vi "Send Command.vi"(8 "error in":errorcluster, 9 "Value":variant, 10 "Command":string, 11 "Electronic Load in":refnum<class "Electronic Load.lvclass">) -> (0 "error out":errorcluster, 3 "Electronic Load out":refnum<class "Electronic Load.lvclass">)   [LabVIEW 2019, in "Electronic Load.lvlib" / "Electronic Load.lvclass"]
uses:
  Library/Electronic Load.lvclass
  C:/Users/Public/Documents/Development/builds/Engine/Engine.lvlibp/Project/Engine.lvclass
  Electronic Load Messages/Write OCP Delay Msg/Write OCP Delay Msg.lvclass/Write OCP Delay Msg.ctl
  Electronic Load Messages/Write OCP Enable Msg/Write OCP Enable Msg.lvclass/Write OCP Enable Msg.ctl
  Electronic Load Messages/Write OCP Level Msg/Write OCP Level Msg.lvclass/Write OCP Level Msg.ctl
  Electronic Load Messages/Write Active Channel Msg/Write Active Channel Msg.lvclass/Write Active Channel Msg.ctl
  Electronic Load Messages/Write Input Level Msg/Write Input Level Msg.lvclass/Write Input Level Msg.ctl
  Electronic Load Messages/Write Mode Msg/Write Mode Msg.lvclass/Write Mode Msg.ctl
  Electronic Load Messages/Write Output Enable Msg/Write Output Enable Msg.lvclass/Write Output Enable Msg.ctl
  Electronic Load Messages/Write Slew Rate Msg/Write Slew Rate Msg.lvclass/Write Slew Rate Msg.ctl
  Electronic Load Messages/Write All Pulse Msg/Write All Pulse Msg.lvclass/Write All Pulse Msg.ctl
  Electronic Load Messages/Write Pulse Data Points Msg/Write Pulse Data Points Msg.lvclass/Write Pulse Data Points Msg.ctl
  Electronic Load Messages/Write Pulse Delay Msg/Write Pulse Delay Msg.lvclass/Write Pulse Delay Msg.ctl
  Electronic Load Messages/Write Pulse Enable Msg/Write Pulse Enable Msg.lvclass/Write Pulse Enable Msg.ctl
  Electronic Load Messages/Write Pulse Initial Msg/Write Pulse Initial Msg.lvclass/Write Pulse Initial Msg.ctl
  Electronic Load Messages/Write Pulse Mode Msg/Write Pulse Mode Msg.lvclass/Write Pulse Mode Msg.ctl
  Electronic Load Messages/Write Pulse Sample Interval Msg/Write Pulse Sample Interval Msg.lvclass/Write Pulse Sample Interval Msg.ctl
  Electronic Load Messages/Write Pulse Slew Msg/Write Pulse Slew Msg.lvclass/Write Pulse Slew Msg.ctl
  Electronic Load Messages/Write Pulse Width Msg/Write Pulse Width Msg.lvclass/Write Pulse Width Msg.ctl
  Electronic Load Messages/Write Transient Msg/Write Transient Msg.lvclass/Write Transient Msg.ctl
  builds/Engine/Engine.lvlibp/Accessors/Read Self Q.vi
  builds/Engine/Actor Framework.lvlibp/1abvi3w/vi.lib/ActorFramework/Message Enqueuer/Enqueue.vi
  builds/Engine/Actor Framework.lvlibp/1abvi3w/vi.lib/ActorFramework/Message Enqueuer/Message Enqueuer.lvclass
  Electronic Load Messages/Write OCP Delay Msg/Write OCP Delay Msg.lvclass
  Electronic Load Messages/Write OCP Enable Msg/Write OCP Enable Msg.lvclass
  Electronic Load Messages/Write OCP Level Msg/Write OCP Level Msg.lvclass
  Electronic Load Messages/Write Active Channel Msg/Write Active Channel Msg.lvclass
  Electronic Load Messages/Write Input Level Msg/Write Input Level Msg.lvclass
  Electronic Load Messages/Write Mode Msg/Write Mode Msg.lvclass
  Electronic Load Messages/Write Output Enable Msg/Write Output Enable Msg.lvclass
  Electronic Load Messages/Write Slew Rate Msg/Write Slew Rate Msg.lvclass
  Electronic Load Messages/Write All Pulse Msg/Write All Pulse Msg.lvclass
  Electronic Load Messages/Write Pulse Data Points Msg/Write Pulse Data Points Msg.lvclass
  Electronic Load Messages/Write Pulse Delay Msg/Write Pulse Delay Msg.lvclass
  Electronic Load Messages/Write Pulse Enable Msg/Write Pulse Enable Msg.lvclass
  Electronic Load Messages/Write Pulse Initial Msg/Write Pulse Initial Msg.lvclass
  Electronic Load Messages/Write Pulse Mode Msg/Write Pulse Mode Msg.lvclass
  Electronic Load Messages/Write Pulse Sample Interval Msg/Write Pulse Sample Interval Msg.lvclass
  Electronic Load Messages/Write Pulse Slew Msg/Write Pulse Slew Msg.lvclass
  Electronic Load Messages/Write Pulse Width Msg/Write Pulse Width Msg.lvclass
  Electronic Load Messages/Write Transient Msg/Write Transient Msg.lvclass
  Electronic Load Messages/Reset Eload Msg/Reset Eload Msg.lvclass
  builds/Instruments/Instruments.lvlibp/Instruments Messages/Take Snapshot Msg/Take Snapshot Msg.lvclass
  builds/Instruments/Instruments.lvlibp/Instruments Messages/Power Off Msg/Power Off Msg.lvclass
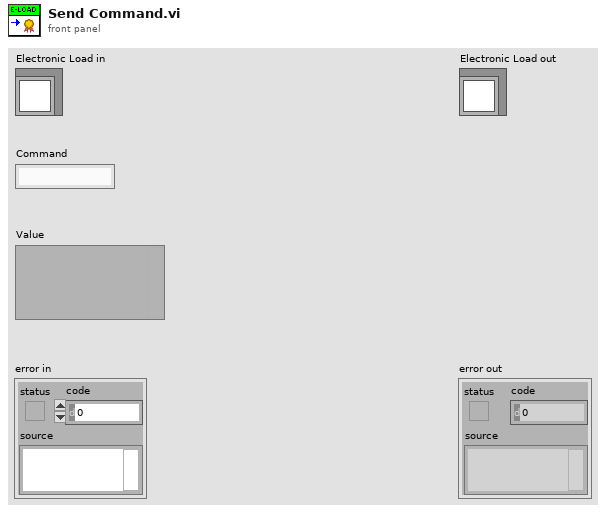
[diagram p1: front panel]
types:
  T1 = typedef "Electronic Load.lvlib/Electronic Load.lvclass/E-Load Mode.ctl" = enum16{"Current", "Resistance", "Voltage"}
  T2 = typedef "Electronic Load.lvlib/Electronic Load.lvclass/Trigger Settings.ctl" = cluster{"Mode":T1, "Initial":dbl, "Transient":dbl, "Interval":dbl, "Width":dbl, "Delay":dbl, "Data Pts":i32, "Slew Rate":dbl}
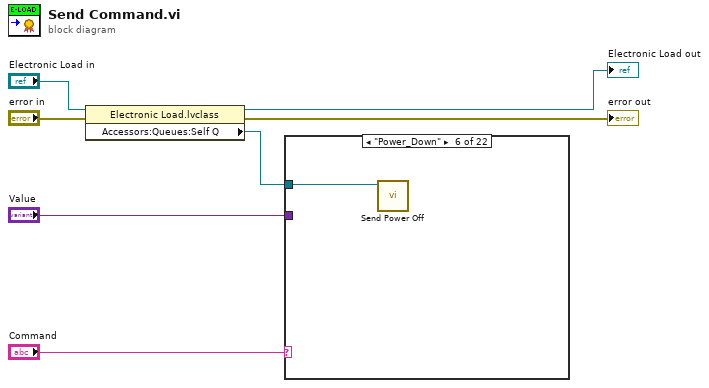
[diagram p0: block diagram]
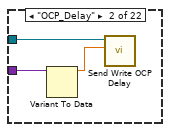
[diagram p3: hidden frame]
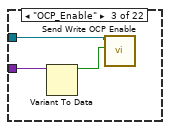
[diagram p4: hidden frame]
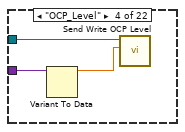
[diagram p5: hidden frame]
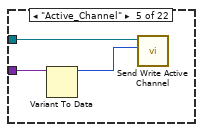
[diagram p6: hidden frame]
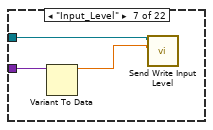
[diagram p7: hidden frame]
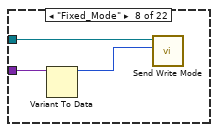
[diagram p8: hidden frame]
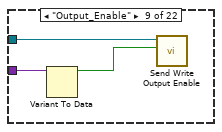
[diagram p9: hidden frame]
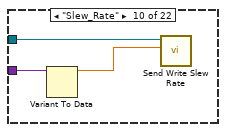
[diagram p10: hidden frame]
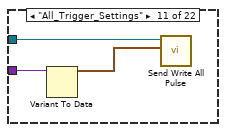
[diagram p11: hidden frame]
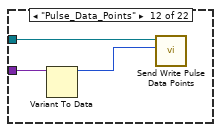
[diagram p12: hidden frame]
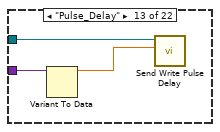
[diagram p13: hidden frame]
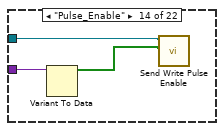
[diagram p14: hidden frame]
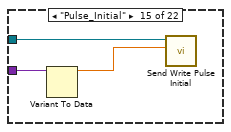
[diagram p15: hidden frame]
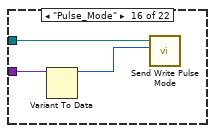
[diagram p16: hidden frame]
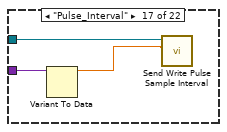
[diagram p17: hidden frame]
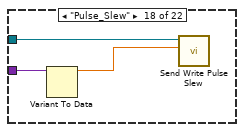
[diagram p18: hidden frame]
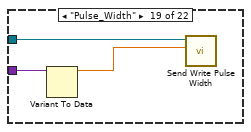
[diagram p19: hidden frame]
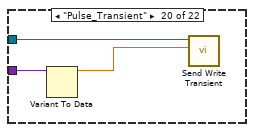
[diagram p20: hidden frame]
diagram:
  n1 = property class="Electronic Load.lvclass"(reference="Electronic Load in", error in="error in") -> (reference out=→"Electronic Load out":refnum<class "Electronic Load.lvclass">, error out=→"error out":errorcluster, "Accessors:Queues:Self Q"=w1:refnum<class "Message Enqueuer.lvclass">)
  n2 = case shown="\"Power_Down\"" "Command" {
    tunnel: "Value" -> [_ w9 w13 w16 w19 _ w23 w26 w29 w32 w35 w38 w41 w44 w47 w50 w53 w56 w59 w62 _ _]
    tunnel: w1 -> [_ w10 w12 w15 w18 w20 w22 w25 w28 w31 w34 w37 w40 w43 w46 w49 w52 w55 w58 w61 w63 w64]
    frame "False", Default {
    }
    frame "OCP_Delay" {
      n3 = Variant To Data(Variant=w9) -> (data=w8:dbl)  [unwired: 2 in, 1 out]
      n4 = call "Send Write OCP Delay.vi"("Delay"=w8, "Message Enqueuer"=w10) -> ()  [unwired: 8 in, 2 out]
    }
    frame "OCP_Enable" {
      n5 = Variant To Data(Variant=w13) -> (data=w11:bool)  [unwired: 2 in, 1 out]
      n6 = call "Send Write OCP Enable.vi"("OCP Enable"=w11, "Message Enqueuer"=w12) -> ()  [unwired: 8 in, 2 out]
    }
    frame "OCP_Level" {
      n7 = Variant To Data(Variant=w16) -> (data=w14:dbl)  [unwired: 2 in, 1 out]
      n8 = call "Send Write OCP Level.vi"("OCP Level"=w14, "Message Enqueuer"=w15) -> ()  [unwired: 8 in, 2 out]
    }
    frame "Active_Channel" {
      n9 = Variant To Data(Variant=w19) -> (data=w17:u32)  [unwired: 2 in, 1 out]
      n10 = call "Send Write Active Channel.vi"("Active Channel"=w17, "Message Enqueuer"=w18) -> ()  [unwired: 8 in, 2 out]
    }
    frame "Power_Down" {
      n11 = call "Send Power Off.vi"("Message Enqueuer"=w20) -> ()  [unwired: 9 in, 2 out]
    }
    frame "Input_Level" {
      n12 = Variant To Data(Variant=w23) -> (data=w21:dbl)  [unwired: 2 in, 1 out]
      n13 = call "Send Write Input Level.vi"("Input Level"=w21, "Message Enqueuer"=w22) -> ()  [unwired: 8 in, 2 out]
    }
    frame "Fixed_Mode" {
      n14 = Variant To Data(Variant=w26) -> (data=w24:T1)  [unwired: 2 in, 1 out]
      n15 = call "Send Write Mode.vi"("Mode"=w24, "Message Enqueuer"=w25) -> ()  [unwired: 8 in, 2 out]
    }
    frame "Output_Enable" {
      n16 = Variant To Data(Variant=w29) -> (data=w27:bool)  [unwired: 2 in, 1 out]
      n17 = call "Send Write Output Enable.vi"("Output"=w27, "Message Enqueuer"=w28) -> ()  [unwired: 8 in, 2 out]
    }
    frame "Slew_Rate" {
      n18 = Variant To Data(Variant=w32) -> (data=w30:dbl)  [unwired: 2 in, 1 out]
      n19 = call "Send Write Slew Rate.vi"("Slew Rate"=w30, "Message Enqueuer"=w31) -> ()  [unwired: 8 in, 2 out]
    }
    frame "All_Trigger_Settings" {
      n20 = Variant To Data(Variant=w35) -> (data=w33:T2)  [unwired: 2 in, 1 out]
      n21 = call "Send Write All Pulse.vi"("Trigger Settings All"=w33, "Message Enqueuer"=w34) -> ()  [unwired: 8 in, 2 out]
    }
    frame "Pulse_Data_Points" {
      n22 = Variant To Data(Variant=w38) -> (data=w36:i32)  [unwired: 2 in, 1 out]
      n23 = call "Send Write Pulse Data Points.vi"("Data Pts"=w36, "Message Enqueuer"=w37) -> ()  [unwired: 8 in, 2 out]
    }
    frame "Pulse_Delay" {
      n24 = Variant To Data(Variant=w41) -> (data=w39:dbl)  [unwired: 2 in, 1 out]
      n25 = call "Send Write Pulse Delay.vi"("Delay"=w39, "Message Enqueuer"=w40) -> ()  [unwired: 8 in, 2 out]
    }
    frame "Pulse_Enable" {
      n26 = Variant To Data(Variant=w44) -> (data=w42:bool[])  [unwired: 2 in, 1 out]
      n27 = call "Send Write Pulse Enable.vi"("Chan_Trig_En"=w42, "Message Enqueuer"=w43) -> ()  [unwired: 8 in, 2 out]
    }
    frame "Pulse_Initial" {
      n28 = Variant To Data(Variant=w47) -> (data=w45:dbl)  [unwired: 2 in, 1 out]
      n29 = call "Send Write Pulse Initial.vi"("Pulse Initial"=w45, "Message Enqueuer"=w46) -> ()  [unwired: 8 in, 2 out]
    }
    frame "Pulse_Mode" {
      n30 = Variant To Data(Variant=w50) -> (data=w48:T1)  [unwired: 2 in, 1 out]
      n31 = call "Send Write Pulse Mode.vi"("Pulse Mode"=w48, "Message Enqueuer"=w49) -> ()  [unwired: 8 in, 2 out]
    }
    frame "Pulse_Interval" {
      n32 = Variant To Data(Variant=w53) -> (data=w51:dbl)  [unwired: 2 in, 1 out]
      n33 = call "Send Write Pulse Sample Interval.vi"("Sample Interval"=w51, "Message Enqueuer"=w52) -> ()  [unwired: 8 in, 2 out]
    }
    frame "Pulse_Slew" {
      n34 = Variant To Data(Variant=w56) -> (data=w54:dbl)  [unwired: 2 in, 1 out]
      n35 = call "Send Write Pulse Slew.vi"("Slew"=w54, "Message Enqueuer"=w55) -> ()  [unwired: 8 in, 2 out]
    }
    frame "Pulse_Width" {
      n36 = Variant To Data(Variant=w59) -> (data=w57:dbl)  [unwired: 2 in, 1 out]
      n37 = call "Send Write Pulse Width.vi"("Pulse Width"=w57, "Message Enqueuer"=w58) -> ()  [unwired: 8 in, 2 out]
    }
    frame "Pulse_Transient" {
      n38 = Variant To Data(Variant=w62) -> (data=w60:dbl)  [unwired: 2 in, 1 out]
      n39 = call "Send Write Transient.vi"("Transient"=w60, "Message Enqueuer"=w61) -> ()  [unwired: 8 in, 2 out]
    }
    frame "Reset" {
      n40 = call "Send Reset Eload.vi"("Message Enqueuer"=w63) -> ()  [unwired: 9 in, 2 out]
    }
    frame "Send_Trigger" {
      n41 = call "Send Take Snapshot.vi"("Message Enqueuer"=w64) -> ()  [unwired: 9 in, 2 out]
    }
  }
